vi "Init.vi"(8 "error in (no error)":errorcluster, 9 "Replication Rounds":u32, 10 "Size":i32) -> (0 "error out":errorcluster, 3 "Map out":refnum<class "Map.lvclass">)   [LabVIEW 2020, in "SquareBattle.lvlib" / "Map.lvclass"]
uses:
  Map.lvclass
  Map.lvclass/Map.ctl
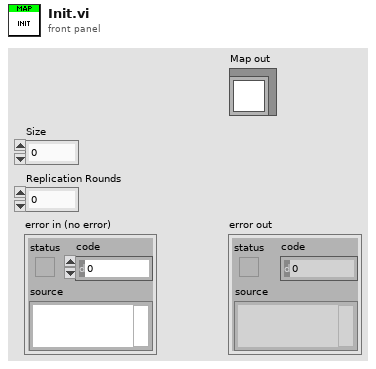
[diagram p1: front panel]
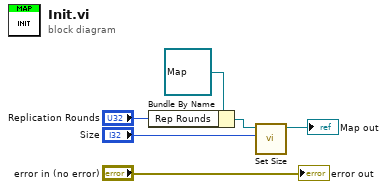
[diagram p0: block diagram]
diagram:
  n1 = Bundle By Name(cluster=refnum<class "Map.lvclass"> refnum ("Map in"), "Rep Rounds"="Replication Rounds") -> (w3:refnum<class "Map.lvclass">)
  n2 = call "Set Size.vi"("Size"="Size", "Map in"=w3) -> ("Map out"=→"Map out":refnum<class "Map.lvclass">)  [unwired: 8 in, 1 out]
  "error out" <- "error in (no error)"
